vi "PEAK-CAN.vi"() -> ()   [LabVIEW 2020]
uses:
  <userlib>/PCANBasic/PCANBasic.lvlib
panel:
  out "Array":T1(array[cluster]) {"ID" format="%.0x"; "DATA[6]" format="%.0x"; "DATA[7]" format="%.0x"}
  out "function return":u32 format="%.0x"
  in  "Channel":u16=81 format="%.0x"
  in  "Btr0Btr1":u16=28 format="%x"
  in  "HwType":u8 format="%.0x"
  in  "IOPort":u32=1
  in  "Interrupt":u16=3 format="%.0x"
  # "// Type of PCAN (non plug&play) hardware\n//\n#define PCAN_TYPE_ISA            0x01U  // PCAN-ISA 82C200\n#define PCAN_TYPE_ISA_SJA        0x09U  // PCAN-ISA SJA1000\n#define PCAN_TYPE_ISA_PHYTEC     0x04U  // PHYTEC ISA \n#define PCAN_TYPE_DNG            0x02U  // PCAN-Dongle 82C200\n#define PCAN_TYPE_DNG_EPP        0x03U  // PCAN-Dongle EPP 82C200\n#define PCAN_TYPE_DNG_SJA        0x05U  // PCAN-Dongle SJA1000\n#define PCAN_TYPE_DNG_SJA_EPP    0x06U  // PCAN-Dongle EPP SJA1000"
  # "c#define PCAN_BAUD_1M             0x0014U  //   1 MBit/s\n#define PCAN_BAUD_800K           0x0016U  // 800 kBit/s\n#define PCAN_BAUD_500K           0x001CU  // 500 kBit/s\n#define PCAN_BAUD_250K           0x011CU  // 250 kBit/s\n#define PCAN_BAUD_125K           0x031CU  // 125 kBit/s\n#define PCAN_BAUD_100K           0x432FU  // 100 kBit/s\n#define PCAN_BAUD_95K            0xC34EU  //  95,238 kBit/s\n#define PCAN_BAUD_83K            0x852BU  //  83,333 kBit/s\n#define PCAN_BAUD_50K            0x472FU  //  50 kBit/s\n#define PCAN_BAUD_47K            0x1414U  //  47,619 kBit/s\n#define PCAN_BAUD_33K            0x8B2FU  //  33,333 kBit/s\n#define PCAN_BAUD_20K            0x532FU  //  20 kBit/s\n#define PCAN_BAUD_10K            0x672FU  //  10 kBit/s\n#define PCAN_BAUD_5K             0x7F7FU  //   5 kBit/s"
  # "PCAN message types\n//\n#define PCAN_MESSAGE_STANDARD    0x00U  // The PCAN message is a CAN Standard Frame (11-bit identifier)\n#define PCAN_MESSAGE_RTR         0x01U  // The PCAN message is a CAN Remote-Transfer-Request Frame\n#define PCAN_MESSAGE_EXTENDED    0x02U  // The PCAN message is a CAN Extended Frame (29-bit identifier)\n#define PCAN_MESSAGE_FD          0x04U  // The PCAN message represents a FD frame in terms of CiA Specs\n#define PCAN_MESSAGE_BRS         0x08U  // The PCAN message represents a FD bit rate switch (CAN data at a higher bit rate)\n#define PCAN_MESSAGE_ESI         0x10U  // The PCAN message represents a FD error state indicator(CAN FD transmitter was error active)\n#define PCAN_MESSAGE_STATUS      0x80U  // The PCAN message represents a PCAN status message"
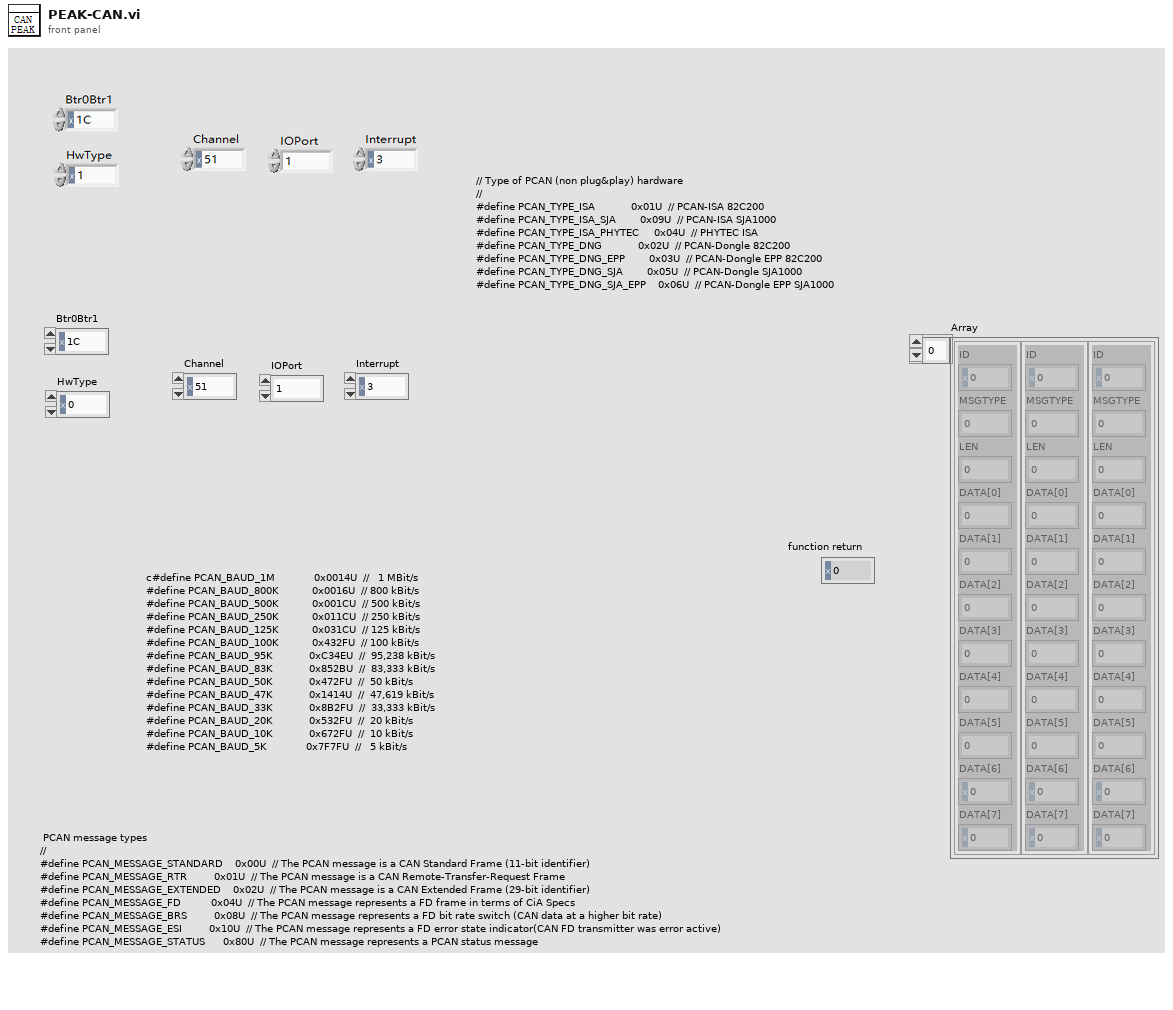
[diagram p1: front panel]
types:
  T1 = cluster{"ID":u32, "MSGTYPE":u8, "LEN":u8, "DATA[0]":u8, "DATA[1]":u8, "DATA[2]":u8, "DATA[3]":u8, "DATA[4]":u8, "DATA[5]":u8, "DATA[6]":u8, "DATA[7]":u8}[]
  T2 = cluster{"ID":u32, "MSGTYPE":u8, "LEN":u8, "DATA[0]":u8, "DATA[1]":u8, "DATA[2]":u8, "DATA[3]":u8, "DATA[4]":u8, "DATA[5]":u8, "DATA[6]":u8, "DATA[7]":u8}
  T3 = cluster{"millis":u32, "millis_overflow":u16, "micros":u16}
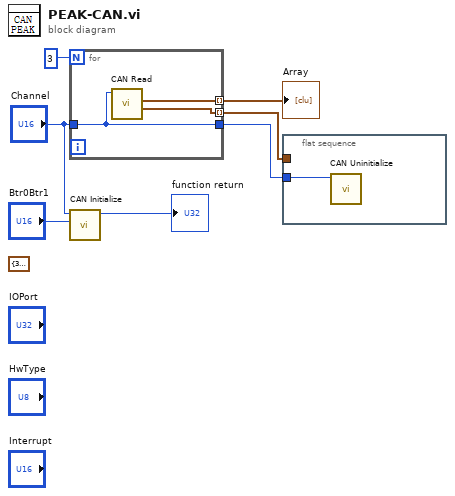
[diagram p0: block diagram]
diagram:
  (unwired) T2 {"ID"=384, "MSGTYPE"=0, "LEN"=8, "DATA[0]"=83, "DATA[1]"=48, "DATA[2]"=48, "DATA[3]"=49, "DATA[4]"=54, "DATA[5]"=57, "DATA[6]"=48, "DATA[7]"=0} ("MessageBuffer")
  n1 = for {
    N: 3 -> [_]
    tunnel: [w10] -> w3 mode=indexing
    tunnel: "Channel" -> [w8]
    tunnel: [w9] -> w4 mode=indexing
    tunnel: [w8] -> w1
    n2 = call <vilib>:"CAN Read.vi"("Channel"=w8) -> ("TimestampBuffer out"=w9:T3, "MessageBuffer out"=w10:T2)  [unwired: 7 in, 2 out]
  }
  "Array" <- w3
  n3 = call <userlib>:"CAN Initialize.vi"("Btr0Btr1"="Btr0Btr1", "Channel"="Channel") -> ("function return"=→"function return":u32)  [unwired: 8 in, 1 out]
  n4 = flat-sequence {
    tunnel: w1 -> [w11]
    tunnel: w4 -> [_]
    frame #0 {
      n5 = call <userlib>:"CAN Uninitialize.vi"("Channel"=w11) -> ()  [unwired: 10 in, 1 out]
    }
  }
